vi "AoA Filter.vi"(10 "IQ Rate":dbl, 11 "Filter":string) -> (0 "B1":dbl[](array[numeric]), 1 "A1":dbl[](array[numeric]), 2 "B2":dbl[](array[numeric]), 3 "A2":dbl[](array[numeric]))   [LabVIEW 2015]
uses:
  <vilib>/imath/engines/lvmath2/RunTimeEngine/BuiltInFunctions/fir_remezord/NIMS_fir_remezord.vi
  <vilib>/imathl/engines/lvmath/Functions/Error Handling/Create Error.vi
  <vilib>/imath/engines/lvmath2/RunTimeEngine/BuiltInFunctions/fir_remez/NIMS_fir_remez().vi
  <vilib>/imath/engines/lvmath2/RunTimeEngine/ErrorHandling/NIMS_Error From Error Code.vi
  <vilib>/imath/engines/lvmath2/RunTimeEngine/NodeEndStatement/NIMS_NodeEndStatement_Output.vi
  <instcachedir>/0/NIMS_NodeEndStatement_Output_53EC0D466D134D7ABD903AC30B43404B.lvgen/NIMS_NodeEndStatement_Output_53EC0D466D134D7ABD903AC30B43404B_004.vi
  <instcachedir>/0/NIMS_NodeEndStatement_Output_53EC0D466D134D7ABD903AC30B43404B.lvgen/NIMS_NodeEndStatement_Output_53EC0D466D134D7ABD903AC30B43404B_005.vi
  <vilib>/imath/engines/lvmath2/RunTimeEngine/ErrorHandling/NIMS_Finalize Error.vi
  <vilib>/Utility/file.llb/Read Delimited Spreadsheet (DBL).vi
  <vilib>/imath/engines/lvmath2/RunTimeEngine/BuiltInFunctions/iir_elliptic/NIMS_[2o]_iir_elliptic(I32,DBL2,V).vi
  <vilib>/imath/engines/lvmath2/RunTimeEngine/ErrorHandling/NIMS_Create Error From Enums.vi
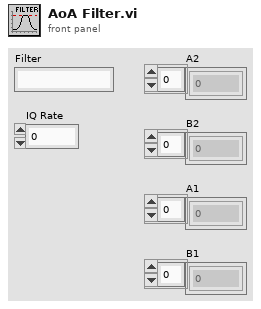
[diagram p1: front panel]
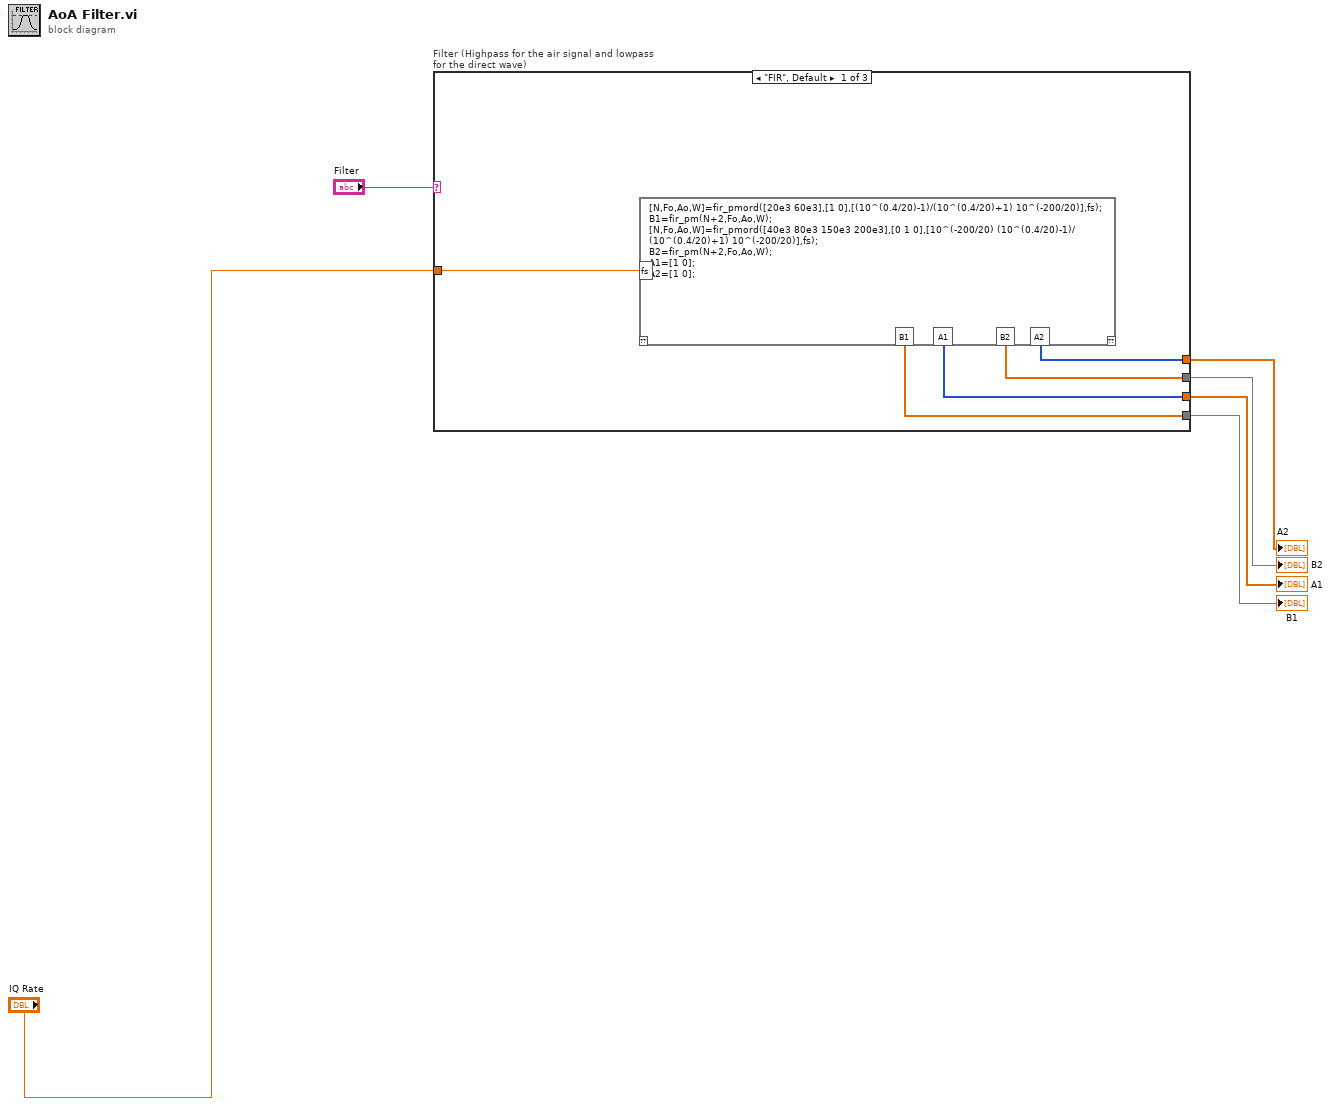
[diagram p0: block diagram]
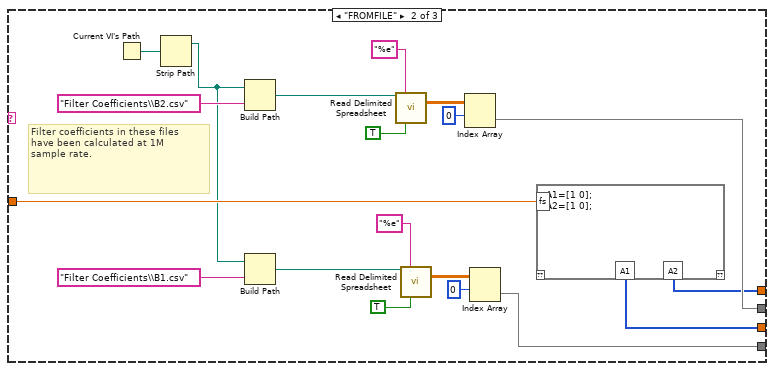
[diagram p2: hidden frame]
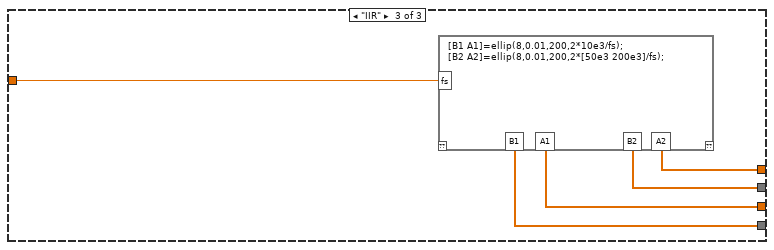
[diagram p3: hidden frame]
diagram:
  n1 = case "Filter (Highpass for the air signal and lowpass for the direct wave)" shown="\"FIR\", Default" "Filter" {
    tunnel: [w11 w194 w225] -> w1
    tunnel: [w7 w182 w222] -> w2
    tunnel: [w10 w189 w224] -> w3
    tunnel: [w8 w181 w221] -> w4
    tunnel: "IQ Rate" -> [w9 w199 w223]
    frame "FIR", Default {
      n2 = mathscript code="[N,Fo,Ao,W]=fir_pmord([20e3 60e3],[1 0],[(10^(0.4/20)-1)/(10^(0.4/20)+1) 10^(-200/20)],fs);\nB1=fir_pm(N+2,Fo,Ao,W);\n[N,Fo,Ao,W]=fir_pmord([40e3 80e3 150e3 200e3],[0 1 0],[10^(-200/20) (10^(0.4/20)-1)/(10^(0.4/20)+1) 10^(-200/20)],fs);\nB2=fir_pm(N+2,Fo,Ao,W);\nA1=[1 0];\nA2=[1 0];"("fs"=w9) -> ("B1"=w11:dbl[], "B2"=w10:dbl[], "A2"=w8:i32[], "A1"=w7:i32[])  [unwired: 1 in, 1 out]
    }
    frame "FROMFILE" {
      # "Filter coefficients in these files\nhave been calculated at 1M\nsample rate."
      n3 = Current VI's Path() -> (path=w188:path)
      n4 = Strip Path(path=w188) -> (stripped path=w184:path)  [unwired: 1 out]
      n5 = Build Path(base path=w184, name or relative path="Filter Coefficients\\B2.csv") -> (appended path=w186:path)
      n6 = Build Path(base path=w184, name or relative path="Filter Coefficients\\B1.csv") -> (appended path=w183:path)
      n7 = call-poly <vilib>:"Read Delimited Spreadsheet.vi"("file path (dialog if empty)"=w186, "format (%.3f)"="%e", "transpose? (F)"=TRUE) -> ("all rows"=w191:dbl[][])  [unwired: 7 in, 5 out]
      n8 = call-poly <vilib>:"Read Delimited Spreadsheet.vi"("file path (dialog if empty)"=w183, "format (%.3f)"="%e", "transpose? (F)"=TRUE) -> ("all rows"=w197:dbl[][])  [unwired: 7 in, 5 out]
      n9 = Index Array(array=w191, index (row)=0) -> (element=w189:dbl[])  [unwired: 1 in]
      n10 = Index Array(array=w197, index (row)=0) -> (element=w194:dbl[])  [unwired: 1 in]
      n11 = mathscript code="A1=[1 0];\nA2=[1 0];"("fs"=w199) -> ("A1"=w182:i32[], "A2"=w181:i32[])  [unwired: 1 in, 1 out]
    }
    frame "IIR" {
      n12 = mathscript code="[B1 A1]=ellip(8,0.01,200,2*10e3/fs);\n[B2 A2]=ellip(8,0.01,200,2*[50e3 200e3]/fs);"("fs"=w223) -> ("B1"=w225:dbl[], "B2"=w224:dbl[], "A1"=w222:dbl[], "A2"=w221:dbl[])  [unwired: 1 in, 1 out]
    }
  }
  "A2" <- w4
  "B2" <- w3
  "A1" <- w2
  "B1" <- w1
